vi "Remove Child.vi"(8 "error in (no error)":errorcluster, 10 "Child":refnum<data-value>, 11 "NodeRef In":refnum<data-value>) -> (0 "error out":errorcluster, 3 "NodeRef":refnum<data-value>)   [LabVIEW 2020, in "PicoG-ParserLexer.lvlib" / "Node.lvclass"]
doc: "Removes <b>Child</b> from the current node's children list.\n\n<b>Error Codes:</b>\n<b>1556</b>: Uninitialized <b>NodeRef In</b> value, Nodes must be initialized by calling Ctor.\n<b>15</b>: The <b>Child</b> was not found as a child of this node."
uses:
  Node.lvclass
  <vilib>/ErrorRing/Error Ring.xnode
  <vilib>/Utility/error.llb/Error Cluster From Error Code.vi
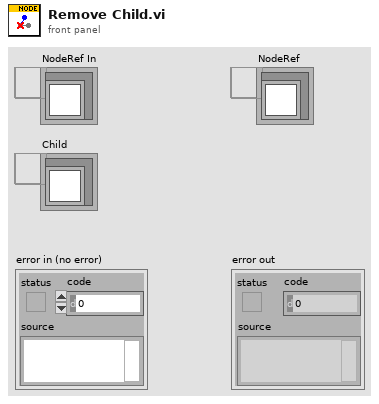
[diagram p1: front panel]
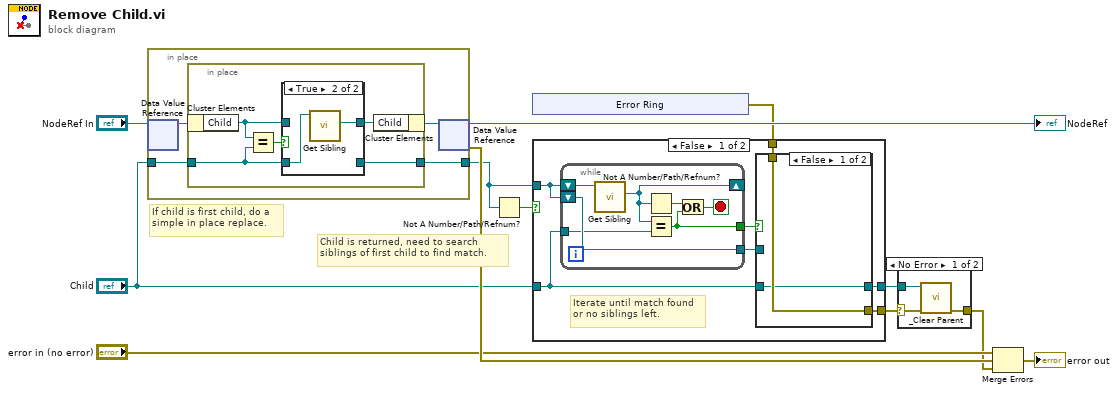
[diagram p0: block diagram]
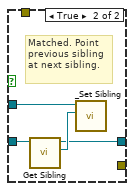
[diagram p3: hidden frame]
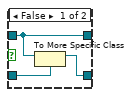
[diagram p5: hidden frame]
diagram:
  # "Child is returned, need to search siblings of first child to find match."
  # "If child is first child, do a simple in place replace."
  n1 = in-place {
    in-place-border: "Child" -> [w16]
    in-place-border: [w13] -> w7
    n2 = in-place-dvr #1("NodeRef In") -> (w15:refnum<class "Node.lvclass">)  [unwired: 1 out]
    n3 = in-place {
      in-place-border: w16 -> [w21]
      in-place-border: [w17] -> w13
      n4 = in-place-cluster #2(w15) -> ("Child"=w19:refnum<data-value>)
      n5 = Equal?(x=w19, y=w21) -> (x = y?=w20:bool)
      n6 = case shown="True" w20 {
        tunnel: w21 -> [w23 w26]
        tunnel: w19 -> [w24 _]
        tunnel: [w24 w25] -> w18
        tunnel: [w22 _] -> w17
        frame False {
          n7 = To More Specific Class(target class=w23, reference=w24) -> (specific class reference=w22:refnum<data-value>)  [unwired: 1 in, 1 out]
        }
        frame True {
          n8 = call "Get Sibling.vi"("NodeRef In"=w26) -> ("Sibling"=w25:refnum<data-value>)  [unwired: 8 in, 2 out]
        }
      }
      n9 = in-place-cluster #2("Child"=w18) -> (w14:refnum<class "Node.lvclass">)
    }
    n10 = in-place-dvr #1(w14) -> (→"NodeRef":refnum<data-value>, w12:errorcluster)
  }
  n11 = Not A Number/Path/Refnum?(number/path/refnum=w7) -> (NaN/Path/Refnum?=w8:bool)
  n12 = xnode "Error Ring"() -> ("error out"=w5:errorcluster)
  n13 = case shown="False" w8 {
    tunnel: w7 -> [w28 _]
    tunnel: "Child" -> [w31 w47]
    tunnel: w5 -> [w30 _]
    tunnel: [w29 _] -> w2
    tunnel: [w27 w47] -> w3
    frame False {
      # "Iterate until match found or no siblings left."
      n14 = while {
        shift-right: [w44] -> _
        shift-left: w28 -> [w46]
        tunnel: w31 -> [w43]
        shift-left: w28 -> [w45]
        tunnel: [w45] -> w32
        tunnel: [w40] -> w33
        stop <- w41 stop-if-true
        n15 = call "Get Sibling.vi"("NodeRef In"=w46) -> ("Sibling"=w44:refnum<data-value>)  [unwired: 8 in, 2 out]
        n16 = Not A Number/Path/Refnum?(number/path/refnum=w44) -> (NaN/Path/Refnum?=w42:bool)
        n17 = Equal?(x=w44, y=w43) -> (x = y?=w40:bool)
        n18 = Or(x=w42, y=w40) -> (x .or. y?=w41:bool)
      }
      n19 = case shown="False" w33 {
        tunnel: w32 -> [_ w38]
        tunnel: w31 -> [w34 w39]
        tunnel: w30 -> [w35 _]
        tunnel: [w35 _] -> w29
        tunnel: [w34 w36] -> w27
        frame False {
        }
        frame True {
          # "Matched. Point previous sibling at next sibling."
          n20 = call "Get Sibling.vi"("NodeRef In"=w39) -> ("Sibling"=w37:refnum<data-value>, "NodeRef"=w36:refnum<data-value>)  [unwired: 8 in, 1 out]
          n21 = call "_Set Sibling.vi"("Sibling"=w37, "NodeRef In"=w38) -> ()  [unwired: 8 in, 2 out]
        }
      }
    }
    frame True {
    }
  }
  n22 = case shown="No Error" w2 {
    selector: w2 -> [w49 w51]
    tunnel: w3 -> [w50 _]
    tunnel: [w48 w51] -> w1
    frame No Error {
      n23 = call "_Clear Parent.vi"("error in (no error)"=w49, "NodeRef In"=w50) -> ("error out"=w48:errorcluster)  [unwired: 8 in, 1 out]
    }
    frame Error {
    }
  }
  n24 = Merge Errors("error in (no error)", w12, w1) -> (→"error out":errorcluster)
